vi "Close Module.vi"(8 "error in":errorcluster, 9 "Wait for stop?":bool, 11 "Module Admin in":refnum<class "Delacor_lib_QMH_Cloneable Module Admin.lvclass">) -> (0 "error out":errorcluster, 1 "External Launch":bool, 3 "Module Admin out":refnum<class "Delacor_lib_QMH_Cloneable Module Admin.lvclass">)   [LabVIEW 2019, in "Multiple_uC.lvlib"]
doc: "Destroy the Broadcast Events and Request Events (if this was the first instance). Reset flags stored in Module Admin class.\n_____\nBased on Delacor QMH Project Template 5.0.0.82."
uses:
  Multiple_uC.lvlib
  <vilib>/Delacor/Delacor QMH/Libraries/Cloneable Module Admin_class/Delacor_lib_QMH_Cloneable Module Admin.lvclass
  C:/Program Files/National Instruments/LabVIEW 2019/vi.lib/Delacor/Delacor QMH/Libraries/Module Admin_class/Delacor_lib_QMH_Module Admin.lvclass
  <vilib>/Delacor/Delacor QMH/Libraries/Cloneable Module Admin_class/Delacor_lib_QMH_Cloneable Module Admin.lvclass/Delacor_lib_QMH_Cloneable Module Admin.ctl
  <vilib>/Delacor/Delacor QMH/Libraries/Module Admin_class/Delacor_lib_QMH_Module Admin.lvclass/Delacor_lib_QMH_Module Admin.ctl
  <vilib>/Delacor/Delacor QMH/Libraries/Cloneable Module Admin_class/Delacor_lib_QMH_Get First.vi
  <vilib>/Delacor/Delacor QMH/Libraries/Cloneable Module Admin_class/Delacor_lib_QMH_Get Module ID.vi
  <vilib>/Delacor/Delacor QMH/Libraries/Module Admin_class/Delacor_lib_QMH_Get External Launch.vi
  <vilib>/Delacor/Delacor QMH/Libraries/Cloneable Module Admin_class/Delacor_lib_QMH_Get Close Master Reference.vi
  Clone Registration/Clone Registration.lvlib
  VI Reference Management/VI Reference Management.lvlib
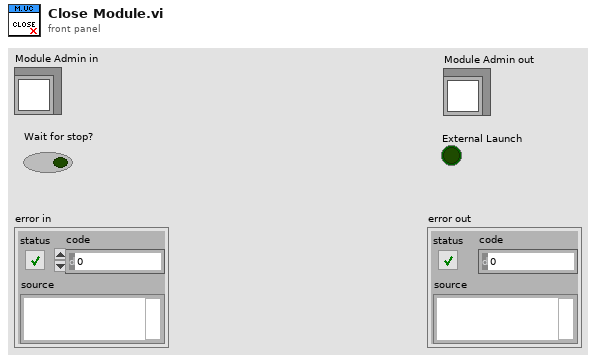
[diagram p1: front panel]
types:
  T1 = typedef "Semaphore RefNum" = refnum<k1>
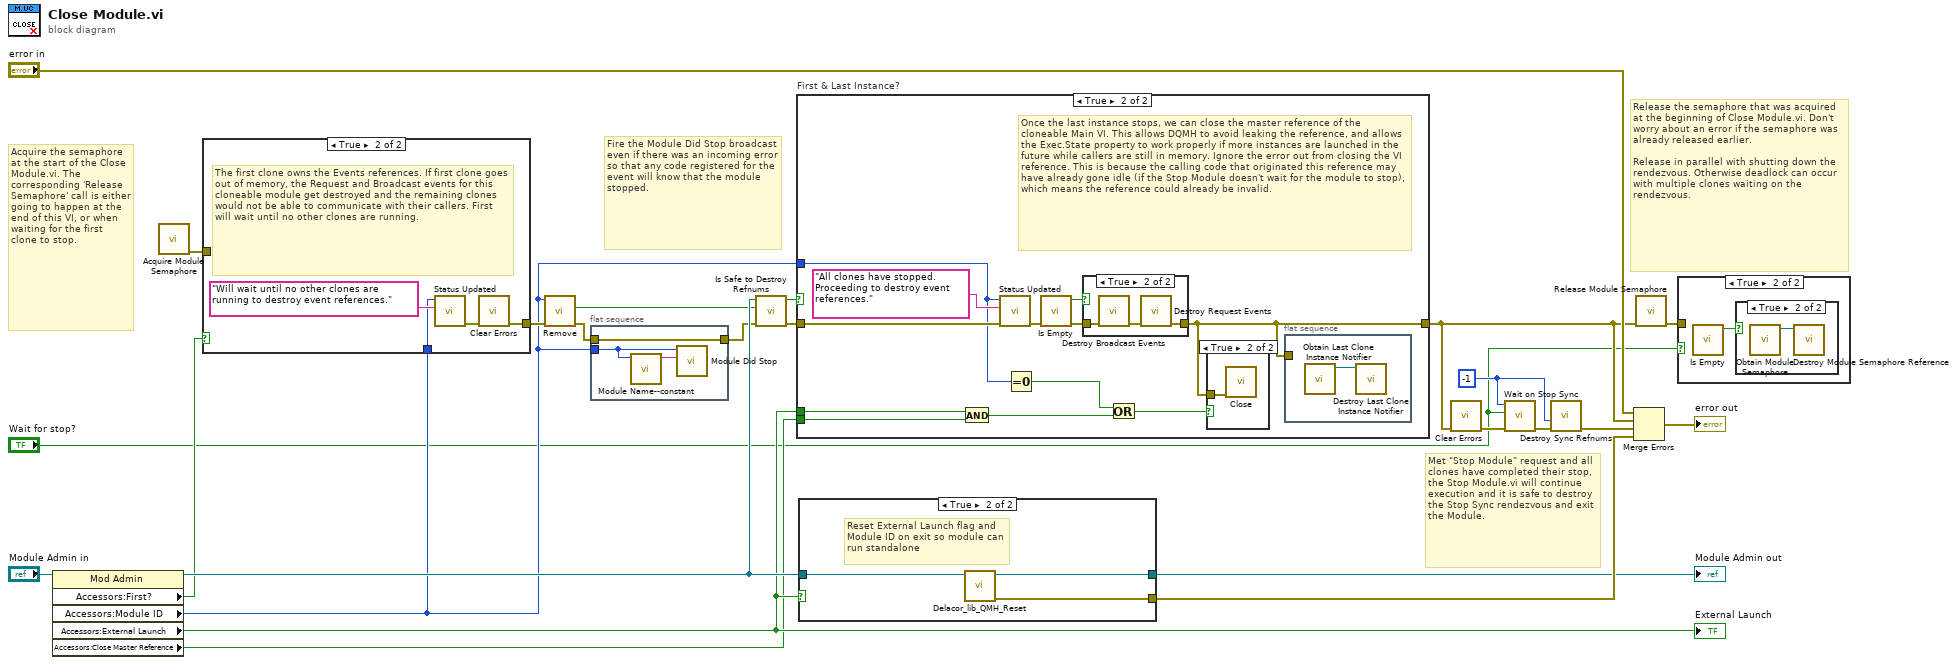
[diagram p0: block diagram]
diagram:
  w15 = -1 ("Module ID")
  # "Release the semaphore that was acquired at the beginning of Close Module.vi. Don't worry about an error if the semaphore was already released earlier.\n\nRelease in parallel with shutting down the rendezvous. Otherwise deadlock can occur with multiple clones waiting on the rendezvous."
  # "Acquire the semaphore at the start of the Close Module.vi. The corresponding 'Release Semaphore' call is either going to happen at the end of this VI, or when waiting for the first clone to stop."
  # "Fire the Module Did Stop broadcast even if there was an incoming error so that any code registered for the event will know that the module stopped."
  # "Met \"Stop Module\" request and all clones have completed their stop, the Stop Module.vi will continue execution and it is safe to destroy the Stop Sync rendezvous and exit the Module."
  n1 = property class="Mod Admin"(reference="Module Admin in") -> (reference out=w22:refnum<class "Delacor_lib_QMH_Cloneable Module Admin.lvclass">, "Accessors:First?"=w13:bool, "Accessors:Module ID"=w7:i32, "Accessors:External Launch"=w11:bool, "Accessors:Close Master Reference"=w6:bool)  [unwired: 1 in, 1 out]
  "External Launch" <- w11
  n2 = call "Acquire Module Semaphore.vi"() -> ("error out"=w5:errorcluster)  [unwired: 11 in]
  n3 = case shown="True" w13 {
    tunnel: w7 -> [_ w27]
    tunnel: [_ w25] -> w24
    tunnel: w5 -> [_ _]
    frame False {
    }
    frame True {
      # "The first clone owns the Events references. If first clone goes out of memory, the Request and Broadcast events for this cloneable module get destroyed and the remaining clones would not be able to communicate with their callers. First will wait until no other clones are running."
      n4 = call "Status Updated.vi"("Status"="Will wait until no other clones are running to destroy event references." ("format string"), "Module ID"=w27) -> ("error out"=w26:errorcluster)  [unwired: 9 in]
      n5 = call <vilib>:"Clear Errors.vi"("error in (no error)"=w26) -> ("error out"=w25:errorcluster)  [unwired: 5 in, 1 out]
    }
  }
  n6 = call "Remove.vi"("error in (no error)"=w24, "Module ID"=w7) -> ("error out"=w9:errorcluster, "empty"=w10:bool)  [unwired: 8 in]
  n7 = flat-sequence {
    tunnel: w9 -> [w31]
    tunnel: [w31] -> w8
    tunnel: w7 -> [w29]
    frame #0 {
      n8 = call "Module Name--constant.vi"("Module ID"=w29) -> ("Module Name"=w30:string)  [unwired: 10 in]
      n9 = call "Module Did Stop.vi"("Origin"=w30, "Module ID"=w29) -> ()  [unwired: 9 in, 1 out]
    }
  }
  n10 = call "Is Safe to Destroy Refnums.vi"("error in"=w8, "empty"=w10, "Module Admin"=w22) -> ("error out"=w19:errorcluster, "Destroy Broadcast & Request Event Refs?"=w20:bool)  [unwired: 7 in]
  n11 = case "First & Last Instance?" shown="True" w20 {
    tunnel: w19 -> [w32 w44]
    tunnel: [w32 w36] -> w3
    tunnel: w7 -> [_ w38]
    tunnel: w11 -> [_ w42]
    tunnel: w6 -> [_ w40]
    frame False {
    }
    frame True {
      # "Once the last instance stops, we can close the master reference of the cloneable Main VI. This allows DQMH to avoid leaking the reference, and allows the Exec.State property to work properly if more instances are launched in the future while callers are still in memory. Ignore the error out from closing the VI reference. This is because the calling code that originated this reference may have already gone idle (if the Stop Module doesn't wait for the module to stop), which means the reference could already be invalid."
      n12 = And(x=w42, y=w40) -> (x .and. y?=w41:bool)
      n13 = call "Status Updated.vi"("error in (no error)"=w44, "Status"="All clones have stopped. Proceeding to destroy event references.", "Module ID"=w38) -> ("error out"=w35:errorcluster)  [unwired: 8 in]
      n14 = Equal To 0?(x=w38) -> (x = 0?=w37:bool)
      n15 = call "Is Empty.vi"("error in (no error)"=w35) -> ("error out"=w34:errorcluster, "Empty?"=w33:bool)  [unwired: 9 in]
      n16 = case shown="True" w33 {
        tunnel: [w45 w47] -> w36
        tunnel: w34 -> [w45 w46]
        frame False {
        }
        frame True {
          n17 = call "Destroy Broadcast Events.vi"("error in (no error)"=w46) -> ("error out"=w48:errorcluster)  [unwired: 10 in]
          n18 = call "Destroy Request Events.vi"("error in (no error)"=w48) -> ("error out"=w47:errorcluster)  [unwired: 10 in]
        }
      }
      n19 = Or(x=w37, y=w41) -> (x .or. y?=w39:bool)
      n20 = case shown="True" w39 {
        tunnel: w36 -> [_ w50]
        frame False {
        }
        frame True {
          n21 = call "Close.vi"("error in (no error)"=w50) -> ()  [unwired: 10 in, 1 out]
        }
      }
      n22 = flat-sequence {
        tunnel: w36 -> [_]
        frame #0 {
          n23 = call "Obtain Last Clone Instance Notifier.vi"() -> ("Last Instance Notifier"=w49:refnum<notifier>)  [unwired: 10 in, 1 out]
          n24 = call "Destroy Last Clone Instance Notifier.vi"("Last Instance Notifier"=w49) -> ()  [unwired: 11 in]
        }
      }
    }
  }
  n25 = case shown="True" w11 {
    tunnel: w22 -> [w51 w54]
    tunnel: [w51 w53] -> w18
    tunnel: [_ w52] -> w23
    frame False {
    }
    frame True {
      # "Reset External Launch flag and Module ID on exit so module can run standalone"
      n26 = call-dynamic "Delacor_lib_QMH_Reset.vi"("Mod Admin in"=w54) -> ("error out"=w52:errorcluster, "Mod Admin out"=w53:refnum<class "Delacor_lib_QMH_Cloneable Module Admin.lvclass">)  [unwired: 9 in]
    }
  }
  "Module Admin out" <- w18
  n27 = call <vilib>:"Clear Errors.vi"("error in (no error)"=w3) -> ("error out"=w14:errorcluster)  [unwired: 5 in, 1 out]
  n28 = call "Wait on Stop Sync.vi"("error in (no error)"=w14, "Wait for Module to stop?"="Wait for stop?", "Module ID"=w15) -> ("error out"=w17:errorcluster)  [unwired: 8 in]
  n29 = call "Destroy Sync Refnums.vi"("error in (no error)"=w17, "Module ID"=w15) -> ("error out"=w16:errorcluster)  [unwired: 9 in]
  n30 = Merge Errors("error in", w3, w16, w23) -> (→"error out":errorcluster)
  n31 = call "Release Module Semaphore.vi"("error in"=w3) -> ("error out"=w2:errorcluster)  [unwired: 10 in]
  n32 = case shown="True" "Wait for stop?" {
    tunnel: w2 -> [_ _]
    frame False {
    }
    frame True {
      n33 = call "Is Empty.vi"() -> ("Empty?"=w55:bool)  [unwired: 10 in, 1 out]
      n34 = case shown="True" w55 {
        frame False {
        }
        frame True {
          n35 = call "Obtain Module Semaphore.vi"() -> ("semaphore"=w56:T1)  [unwired: 9 in, 2 out]
          n36 = call "Destroy Module Semaphore Reference.vi"("semaphore"=w56) -> ()  [unwired: 10 in, 1 out]
        }
      }
    }
  }
